vi "niDTS WLAN INSTR RX Configure Standard Parameters.vi"(8 "error in (no error)":errorcluster, 11 "niDTS WLAN INSTR RX in":refnum<class "niDTS WLAN INSTR RX.lvclass">) -> (0 "error out":errorcluster, 3 "niDTS WLAN INSTR RX out":refnum<class "niDTS WLAN INSTR RX.lvclass">)   [LabVIEW 2015, in "niDTS WLAN.lvlib" / "niDTS WLAN INSTR RX.lvclass"]
doc: "Sets:\n* DataRate\n*McsIndex\n*NumberOfTxChains\n\nMissing:\n* FEC Type\n* Guard Interval"
uses:
  niDTS WLAN INSTR RX.lvclass
  niDTS WLAN INSTR RX.lvclass/niDTS WLAN INSTR RX.ctl
  RiviInstDriver/niRfsgWlan/Objects/niRfsgWlan.lvclass
  niDTS WLAN.lvlib
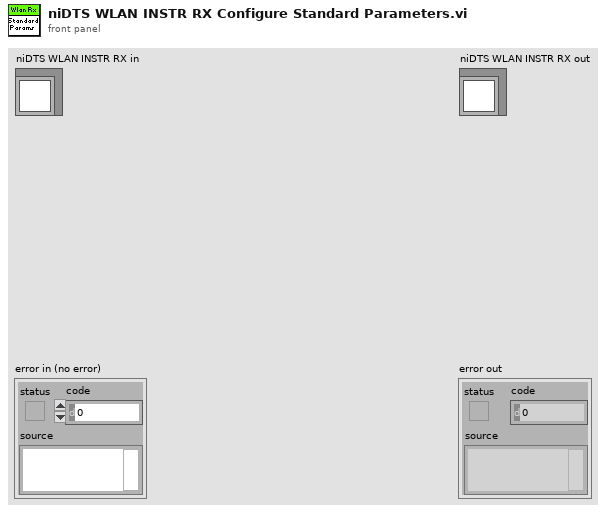
[diagram p1: front panel]
types:
  T1 = enum16{"R1M", "R2M", "R5M5", "R6M", "R9M", "R11M", "R12M", "R18M", "R24M", "R36M", "R48M", "R54M"}
  T2 = typedef "niRfsgWlan.lvclass/niRfsgWlan INC Handle.ctl" = refnum<data-value>
  T3 = typedef "niDTS WLAN.lvlib/niDTS WLAN INC Standard.ctl" = enum16{"802.11 b DSSS", "802.11 a/g OFDM", "802.11 n HT", "802.11 ac VHT"}
  T4 = typedef "niDTS WLAN.lvlib/niDTS WLAN INC DSSS Data Rate.ctl" = enum16{"1", "2", "5.5", "11"}
  T5 = typedef "niDTS WLAN.lvlib/niDTS WLAN INC OFDM Data Rate.ctl" = enum16{"6", "9", "12", "18", "24", "36", "48", "54"}
  T6 = typedef "niDTS WLAN.lvlib/niDTS WLAN INC GI.ctl" = enum16{"LONG", "SHORT"}
  T7 = typedef "niDTS WLAN.lvlib/niDTS WLAN INC FEC Coding.ctl" = enum16{"BCC", "LDPC"}
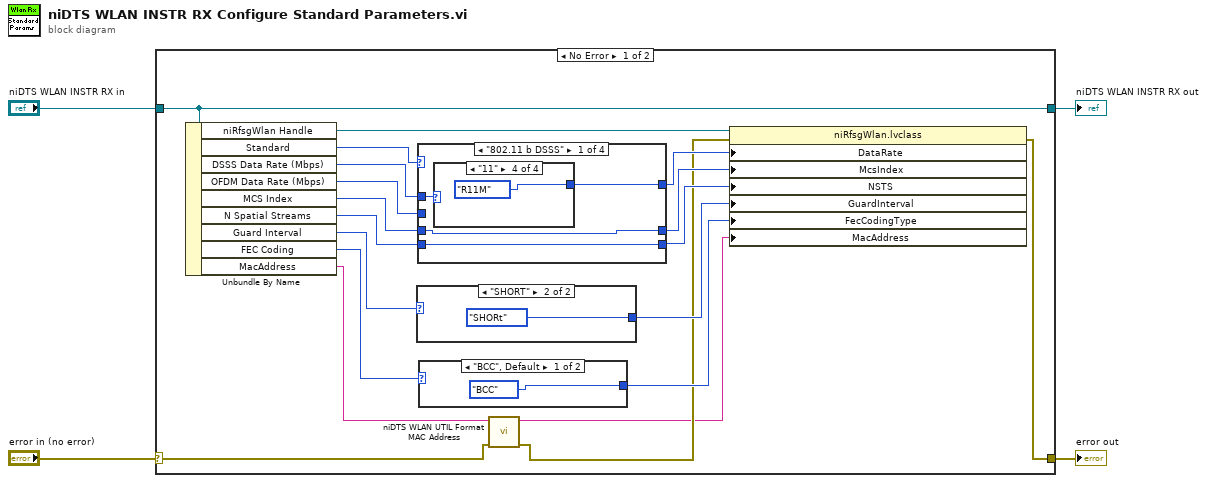
[diagram p0: block diagram]
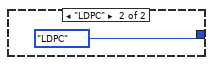
[diagram p2: hidden frame]
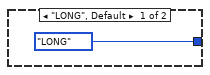
[diagram p3: hidden frame]
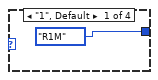
[diagram p4: hidden frame]
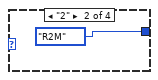
[diagram p5: hidden frame]
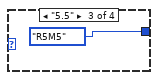
[diagram p6: hidden frame]
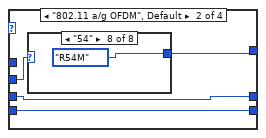
[diagram p7: hidden frame]
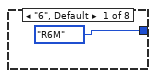
[diagram p8: hidden frame]
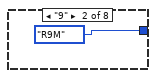
[diagram p9: hidden frame]
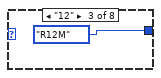
[diagram p10: hidden frame]
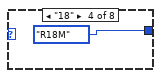
[diagram p11: hidden frame]
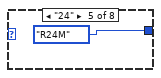
[diagram p12: hidden frame]
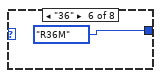
[diagram p13: hidden frame]
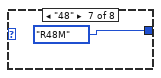
[diagram p14: hidden frame]
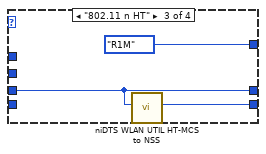
[diagram p15: hidden frame]
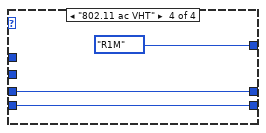
[diagram p16: hidden frame]
diagram:
  n1 = case shown="No Error" "error in (no error)" {
    selector: "error in (no error)" -> [w7 w55]
    tunnel: [w21 w55] -> w3
    tunnel: [w23 w54] -> w1
    tunnel: "niDTS WLAN INSTR RX in" -> [w23 w54]
    frame No Error {
      n2 = Unbundle By Name(w23) -> ("niRfsgWlan Handle"=w22:T2, "Standard"=w20:T3, "DSSS Data Rate (Mbps)"=w19:T4, "OFDM Data Rate (Mbps)"=w18:T5, "MCS Index"=w17:i32, "N Spatial Streams"=w15:i32, "Guard Interval"=w12:T6, "FEC Coding"=w10:T7, "MacAddress"=w8:string)
      n3 = case shown="\"SHORT\"" w12 {
        tunnel: [enum16{"LONG", "SHORt"}."LONG" ("SOURce:RFSG:WLAN:PACKet:GuardInterval") enum16{"LONG", "SHORt"}."SHORt" ("SOURce:RFSG:WLAN:PACKet:GuardInterval")] -> w11
        frame "LONG", Default {
        }
        frame "SHORT" {
        }
      }
      n4 = case shown="\"802.11 b DSSS\"" w20 {
        tunnel: w19 -> [w31 _ _ _]
        tunnel: w18 -> [_ w39 _ _]
        tunnel: [w30 w38 T1."R1M" ("SOURce:RFSG:WLAN:DataRate") T1."R1M" ("SOURce:RFSG:WLAN:DataRate")] -> w13
        tunnel: w17 -> [w29 w36 w50 w53]
        tunnel: [w29 w36 w50 w53] -> w16
        tunnel: [w28 w37 w49 w52] -> w14
        tunnel: w15 -> [w28 w37 _ w52]
        frame "802.11 b DSSS" {
          n5 = case shown="\"11\"" w31 {
            tunnel: [T1."R1M" ("SOURce:RFSG:WLAN:DataRate") T1."R2M" ("SOURce:RFSG:WLAN:DataRate") T1."R5M5" ("SOURce:RFSG:WLAN:DataRate") T1."R11M" ("SOURce:RFSG:WLAN:DataRate")] -> w30
            frame "1", Default {
            }
            frame "2" {
            }
            frame "5.5" {
            }
            frame "11" {
            }
          }
        }
        frame "802.11 a/g OFDM", Default {
          n6 = case shown="\"54\"" w39 {
            tunnel: [T1."R6M" ("SOURce:RFSG:WLAN:DataRate") T1."R9M" ("SOURce:RFSG:WLAN:DataRate") T1."R12M" ("SOURce:RFSG:WLAN:DataRate") T1."R18M" ("SOURce:RFSG:WLAN:DataRate") T1."R24M" ("SOURce:RFSG:WLAN:DataRate") T1."R36M" ("SOURce:RFSG:WLAN:DataRate") T1."R48M" ("SOURce:RFSG:WLAN:DataRate") T1."R54M" ("SOURce:RFSG:WLAN:DataRate")] -> w38
            frame "6", Default {
            }
            frame "9" {
            }
            frame "12" {
            }
            frame "18" {
            }
            frame "24" {
            }
            frame "36" {
            }
            frame "48" {
            }
            frame "54" {
            }
          }
        }
        frame "802.11 n HT" {
          n7 = call "niDTS WLAN UTIL HT-MCS to NSS.vi"("HT MCS"=w50) -> ("NSS"=w49:i32)  [unwired: 10 in]
        }
        frame "802.11 ac VHT" {
        }
      }
      n8 = case shown="\"BCC\", Default" w10 {
        tunnel: [enum16{"BCC", "LDPC"}."BCC" ("SOURce:RFSG:WLAN:PACKet:PAYLoad:FecCodingType") enum16{"BCC", "LDPC"}."LDPC" ("SOURce:RFSG:WLAN:PACKet:PAYLoad:FecCodingType")] -> w9
        frame "BCC", Default {
        }
        frame "LDPC" {
        }
      }
      n9 = call "niDTS WLAN UTIL Format MAC Address.vi"("error in (no error)"=w7, "MAC Address In"=w8) -> ("error out"=w6:errorcluster, "MAC Address Out"=w5:string)  [unwired: 8 in]
      n10 = property class="niRfsgWlan.lvclass"(reference=w22, error in=w6, "DataRate"=w13, "McsIndex"=w16, "NSTS"=w14, "GuardInterval"=w11, "FecCodingType"=w9, "MacAddress"=w5) -> (error out=w21:errorcluster)  [unwired: 1 out]
    }
    frame Error {
    }
  }
  "error out" <- w3
  "niDTS WLAN INSTR RX out" <- w1
